vi "Error Message Handler.vi"(8 "Error In":errorcluster) -> (0 "Error Out":errorcluster, 3 "T button?":bool)   [LabVIEW 2018]
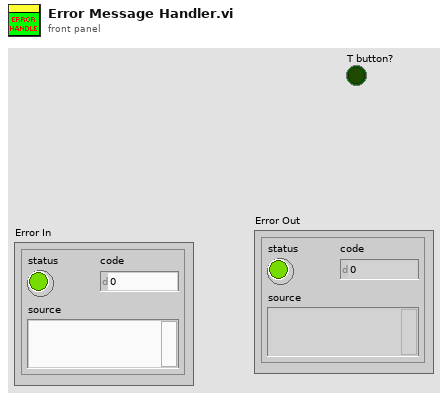
[diagram p1: front panel]
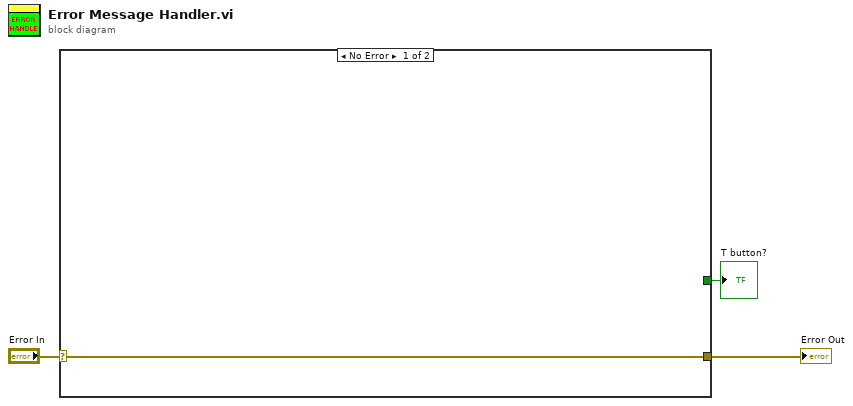
[diagram p0: block diagram]
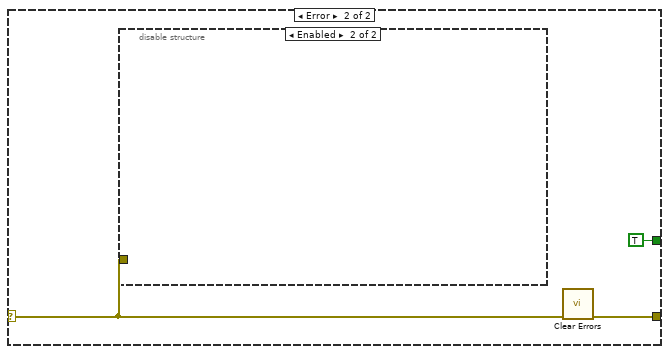
[diagram p2: hidden frame]
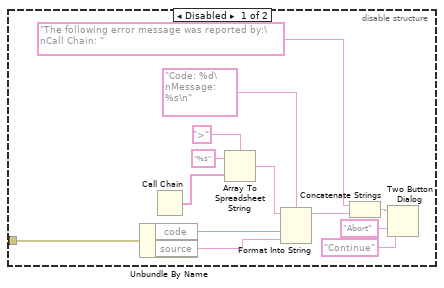
[diagram p3: hidden frame]
diagram:
  n1 = case shown="No Error" "Error In" {
    selector: "Error In" -> [w4 w6]
    tunnel: [w4 w7] -> w2
    tunnel: [_ TRUE ("T button?")] -> w1
    frame No Error {
    }
    frame Error {
      n2 = disable-structure shown="Enabled" {
        disable-tunnel: w6 -> [w19 _]
        frame Disabled {
          n3 = Unbundle By Name(w19) -> ("code"=w18:i32, "source"=w17:string)
          n4 = Call Chain() -> (call chain=w20:string[])
          n5 = Array To Spreadsheet String(delimiter (Tab)=">", array=w20, 3:"%s" ("format string")) -> (spreadsheet string=w15:string)
          n6 = Format Into String(format string="Code: %d\nMessage: %s\n", initial string=w15, w18, w17) -> (resulting string=w14:string)  [unwired: 1 in, 1 out]
          n7 = Concatenate Strings("The following error message was reported by:\nCall Chain: ", w14) -> (w11:string)
          n8 = Two Button Dialog(message=w11, 1:"Continue" ("F button name (\"Cancel\")"), 2:"Abort" ("T button name (\"OK\")")) -> ()  [unwired: 1 out]
        }
        frame Enabled {
        }
      }
      n9 = call <vilib>:"Clear Errors.vi"("error in (no error)"=w6) -> ("error out"=w7:errorcluster)  [unwired: 5 in, 1 out]
    }
  }
  "Error Out" <- w2
  "T button?" <- w1
